vi "Measure - NI 9234.vi"(8 "Error In":errorcluster) -> (0 "Error Out":errorcluster)   [LabVIEW 2011]
uses:
  <vilib>/DAQmx/read.llb/DAQmx Read.vi
  <vilib>/DAQmx/read.llb/DAQmx Read (Analog 1D Wfm NChan NSamp).vi
  <vilib>/DAQmx/miscellaneous.llb/DAQmx Fill In Error Info.vi
panel:
  out "data":waveform(dbl)[](graph) caption="Chart"
  in  "stop":bool
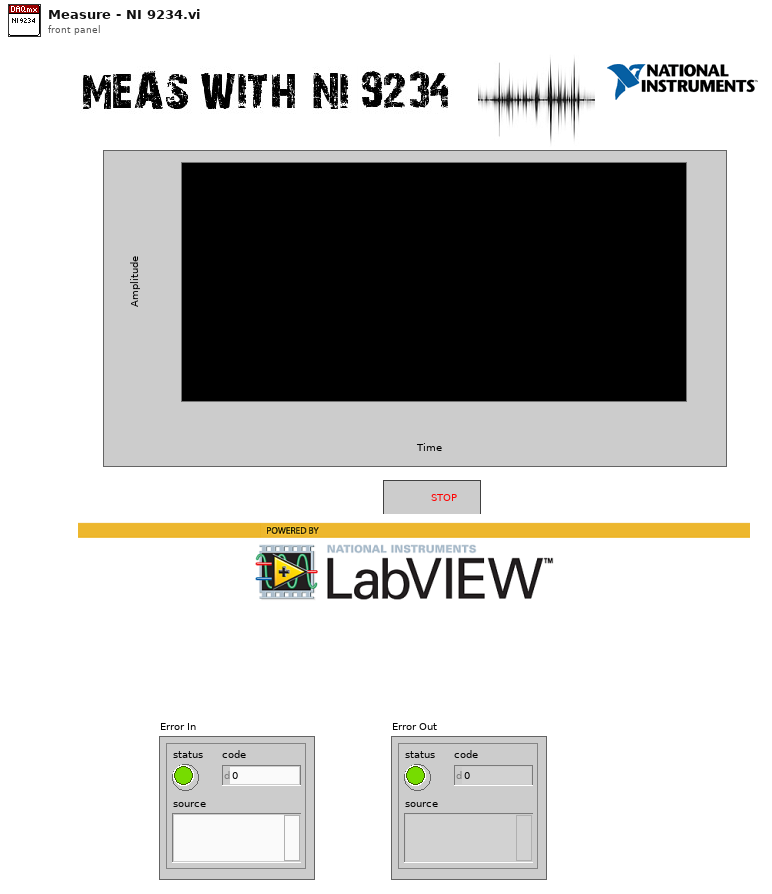
[diagram p1: front panel]
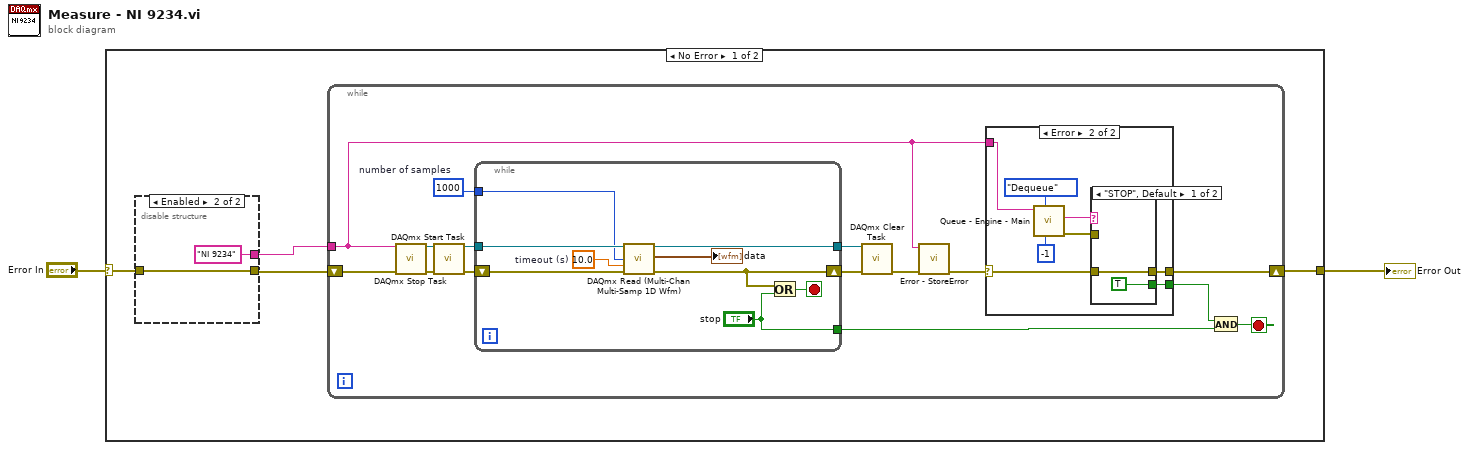
[diagram p0: block diagram]
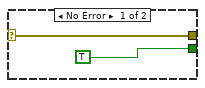
[diagram p2: hidden frame]
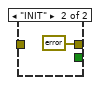
[diagram p3: hidden frame]
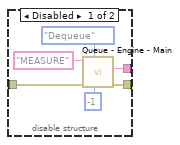
[diagram p4: hidden frame]
diagram:
  n1 = case shown="No Error" "Error In" {
    selector: "Error In" -> [w6 w52]
    tunnel: [w5 w52] -> w2
    frame No Error {
      n2 = disable-structure shown="Enabled" {
        disable-tunnel: [w49 w51] -> w3
        disable-tunnel: [w48 "NI 9234" ("Variable In")] -> w4
        disable-tunnel: w6 -> [w47 w51]
        frame Disabled {
          n3 = call "Queue - Engine - Main.vi"("timeout in ms (-1)"=-1, "Operation"=enum16{"Enqueue", "Dequeue", "Flush", "Release"}."Dequeue", "error in"=w47, "Queue Name In"="MEASURE") -> ("error out"=w49:errorcluster, "Data Out"=w48:string)  [unwired: 5 in, 1 out]
        }
        frame Enabled {
        }
      }
      n4 = while {
        tunnel: w4 -> [w12]
        shift-right: [w11] -> w5
        shift-left: w3 -> [w13]
        stop <- w7 stop-if-true
        w19 = 1000  # number of samples
        n5 = call <vilib>:"DAQmx Stop Task.vi"("task/channels in"=w12, "error in"=w13) -> ("task out"=w16:refnum<k21>, "error out"=w15:errorcluster)  [unwired: 12 in]
        n6 = call <vilib>:"DAQmx Start Task.vi"("task/channels in"=w16, "error in"=w15) -> ("task out"=w21:refnum<k21>, "error out"=w20:errorcluster)  [unwired: 12 out]
        n7 = while {
          tunnel: w21 -> [w43]
          tunnel: w19 -> [w40]
          tunnel: [w41] -> w17
          shift-right: [w38] -> w18
          shift-left: w20 -> [w42]
          tunnel: ["stop"] -> w8
          stop <- w39 stop-if-true
          w37 = 10.0  # timeout (s)
          n8 = call-poly "DAQmx Read (Multi-Chan Multi-Samp 1D Wfm).vi"("task/channels in"=w43, "number of samples per channel"=w40, "timeout"=w37, "error in"=w42) -> ("task out"=w41:refnum<k21>, "data"=→"data":waveform(dbl)[], "error out"=w38:errorcluster)  [unwired: 9 out]
          n9 = Or(x=w38, y="stop") -> (x .or. y?=w39:bool)
        }
        n10 = call <vilib>:"DAQmx Clear Task.vi"("task in"=w17, "error in"=w18) -> ("error out"=w14:errorcluster)  [unwired: 13 out]
        n11 = call "Error - StoreError.vi"("Error In"=w14, "Error Source In"=w12) -> ("Error Out"=w10:errorcluster)  [unwired: 8 in, 1 out]
        n12 = case shown="Error" w10 {
          selector: w10 -> [w23 w24]
          tunnel: [w23 w26] -> w11
          tunnel: [TRUE w25] -> w9
          tunnel: w12 -> [_ w29]
          frame No Error {
          }
          frame Error {
            n13 = call "Queue - Engine - Main.vi"("timeout in ms (-1)"=-1, "Operation"=enum16{"Enqueue", "Dequeue", "Flush", "Release"}."Dequeue", "Queue Name In"=w29) -> ("error out"=w28:errorcluster, "Data Out"=w27:string)  [unwired: 6 in, 1 out]
            n14 = case shown="\"STOP\", Default" w27 {
              tunnel: w28 -> [_ _]
              tunnel: [w32 errorcluster {"status"=FALSE, "code"=0, "source"=""} ("error out")] -> w26
              tunnel: [TRUE _] -> w25
              tunnel: w24 -> [w32 _]
              frame "STOP", Default {
              }
              frame "INIT" {
              }
            }
          }
        }
        n15 = And(x=w9, y=w8) -> (x .and. y?=w7:bool)
      }
    }
    frame Error {
    }
  }
  "Error Out" <- w2
